vi "Dialog Button.vi"() -> ()   [LabVIEW 2020]
panel:
  in  "message":string
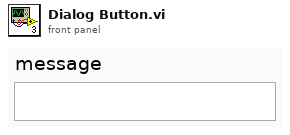
[diagram p1: front panel]
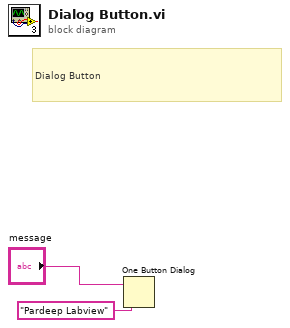
[diagram p0: block diagram]
diagram:
  # "Dialog Button"
  n1 = One Button Dialog(message="message", button name ("OK")="Pardeep Labview") -> ()  [unwired: 1 out]
